vi "Subpanel - Load VI.vi"(7 "SubPanel in":refnum<vi>, 8 "error in (no error)":errorcluster, 10 "Full Delimited Name":string, 11 "Subpanel VI Ref IN":refnum<vi>) -> (0 "error out":errorcluster, 2 "Path to  removed VI":path, 3 "Subpanel VI Ref OUT":refnum<vi>)   [LabVIEW 2014, in "hse-ui.lvlib"]
doc: "Opens the VI reference to <b>Full Delimited Name</b> and inserts it into <b>SubPanel in</b>. The reference of the inserted VI is returned in Subpanel VI Ref OUT.\n\nIf Subpanel VI Ref IN is a valid reference, the front panel of the referenced VI is opened hidden before removing it from the subpanel in order to avoid losing the VI from memory."
uses:
  hse-ui.lvlib
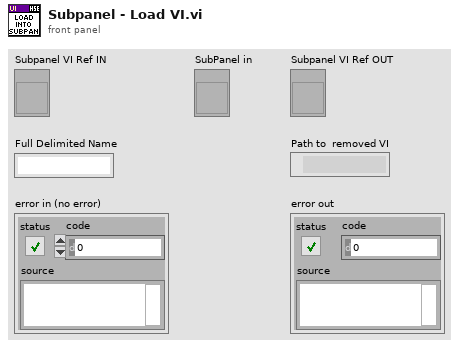
[diagram p1: front panel]
types:
  T1 = enum32{"Invalid", "Standard", "Closed", "Hidden", "Minimized", "Maximized"}
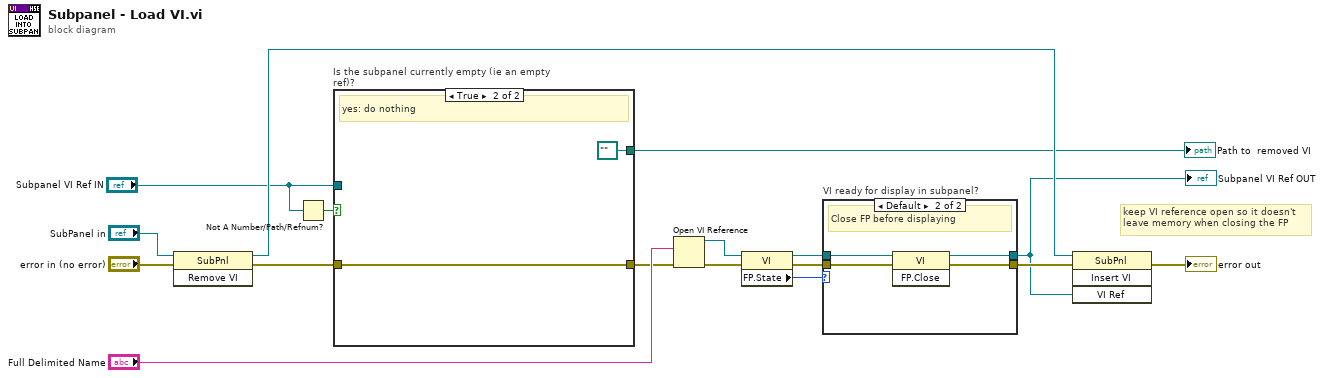
[diagram p0: block diagram]
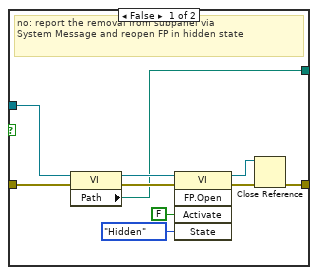
[diagram p2: hidden frame]
diagram:
  # "keep VI reference open so it doesn't\nleave memory when closing the FP"
  n1 = invoke on="Invoke Node" class="SubPnl" method="Remove VI"(reference="SubPanel in", error in="error in (no error)") -> (reference out=w10:refnum<vi>, error out=w5:errorcluster)  [unwired: 1 in, 1 out]
  n2 = Not A Number/Path/Refnum?(number/path/refnum="Subpanel VI Ref IN") -> (NaN/Path/Refnum?=w2:bool)
  n3 = case "Is the subpanel currently empty (ie an empty ref)?" shown="True" w2 {
    tunnel: w5 -> [w20 w29]
    tunnel: [w26 w29] -> w4
    tunnel: "Subpanel VI Ref IN" -> [w22 _]
    tunnel: [w18 path "" ("Path")] -> w1
    frame False {
      # "no: report the removal from subpanel via \nSystem Message and reopen FP in hidden state"
      n4 = property class="VI"(reference=w22, error in=w20) -> (reference out=w21:refnum<vi>, error out=w19:errorcluster, "Path"=w18:path)
      n5 = invoke on="Invoke Node" class="VI" method="FP.Open"(reference=w21, error in=w19, "Activate"=FALSE ("Activate?"), "State"=T1."Hidden") -> (reference out=w25:refnum<vi>, error out=w27:errorcluster)  [unwired: 1 in, 3 out]
      n6 = Close Reference(reference=w25, error in (no error)=w27) -> (error out=w26:errorcluster)
    }
    frame True {
      # "yes: do nothing"
    }
  }
  "Path to  removed VI" <- w1
  n7 = Open VI Reference(vi path="Full Delimited Name", error in (no error)=w4) -> (vi reference=w16:refnum<vi>, error out=w12:errorcluster)  [unwired: 4 in]
  n8 = property class="VI"(reference=w16, error in=w12) -> (reference out=w14:refnum<vi>, error out=w13:errorcluster, "FP.State"=w9:T1)
  n9 = case "VI ready for display in subpanel?" shown="Default" w9 {
    tunnel: w14 -> [w31 w35]
    tunnel: w13 -> [w30 w34]
    tunnel: [w30 w33] -> w11
    tunnel: [w31 w32] -> w7
    frame "Invalid", "Closed" {
      # "state allows display in subpanel"
    }
    frame Default {
      # "Close FP before displaying"
      n10 = invoke on="Invoke Node" class="VI" method="FP.Close"(reference=w35, error in=w34) -> (reference out=w32:refnum<vi>, error out=w33:errorcluster)  [unwired: 1 in, 1 out]
    }
  }
  "Subpanel VI Ref OUT" <- w7
  n11 = invoke on="Invoke Node" class="SubPnl" method="Insert VI"(reference=w10, error in=w11, "VI Ref"=w7) -> (error out=→"error out":errorcluster)  [unwired: 1 in, 3 out]
